vi "传感器测试单片译码器.vi"() -> ()   [LabVIEW 2018]
panel:
  out "缓存":dbl
  out "数值 2":dbl
  out "data 6":bool[](array[boolean]) caption="数据"
  out "初始化的数组 2":dbl[][](array[numeric])
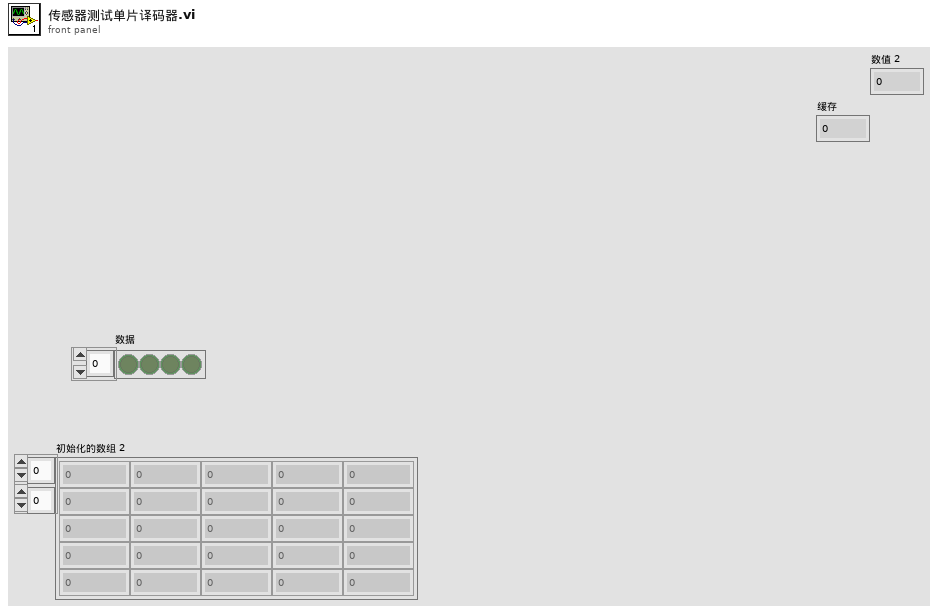
[diagram p1: front panel]
types:
  T1 = enum16{"初始化", "s11", "s12", "s13", "s14", "s15", "s21", "s22", "s23", "s24", "s25", "s31", "s32", "s33", "s34", "s35"}
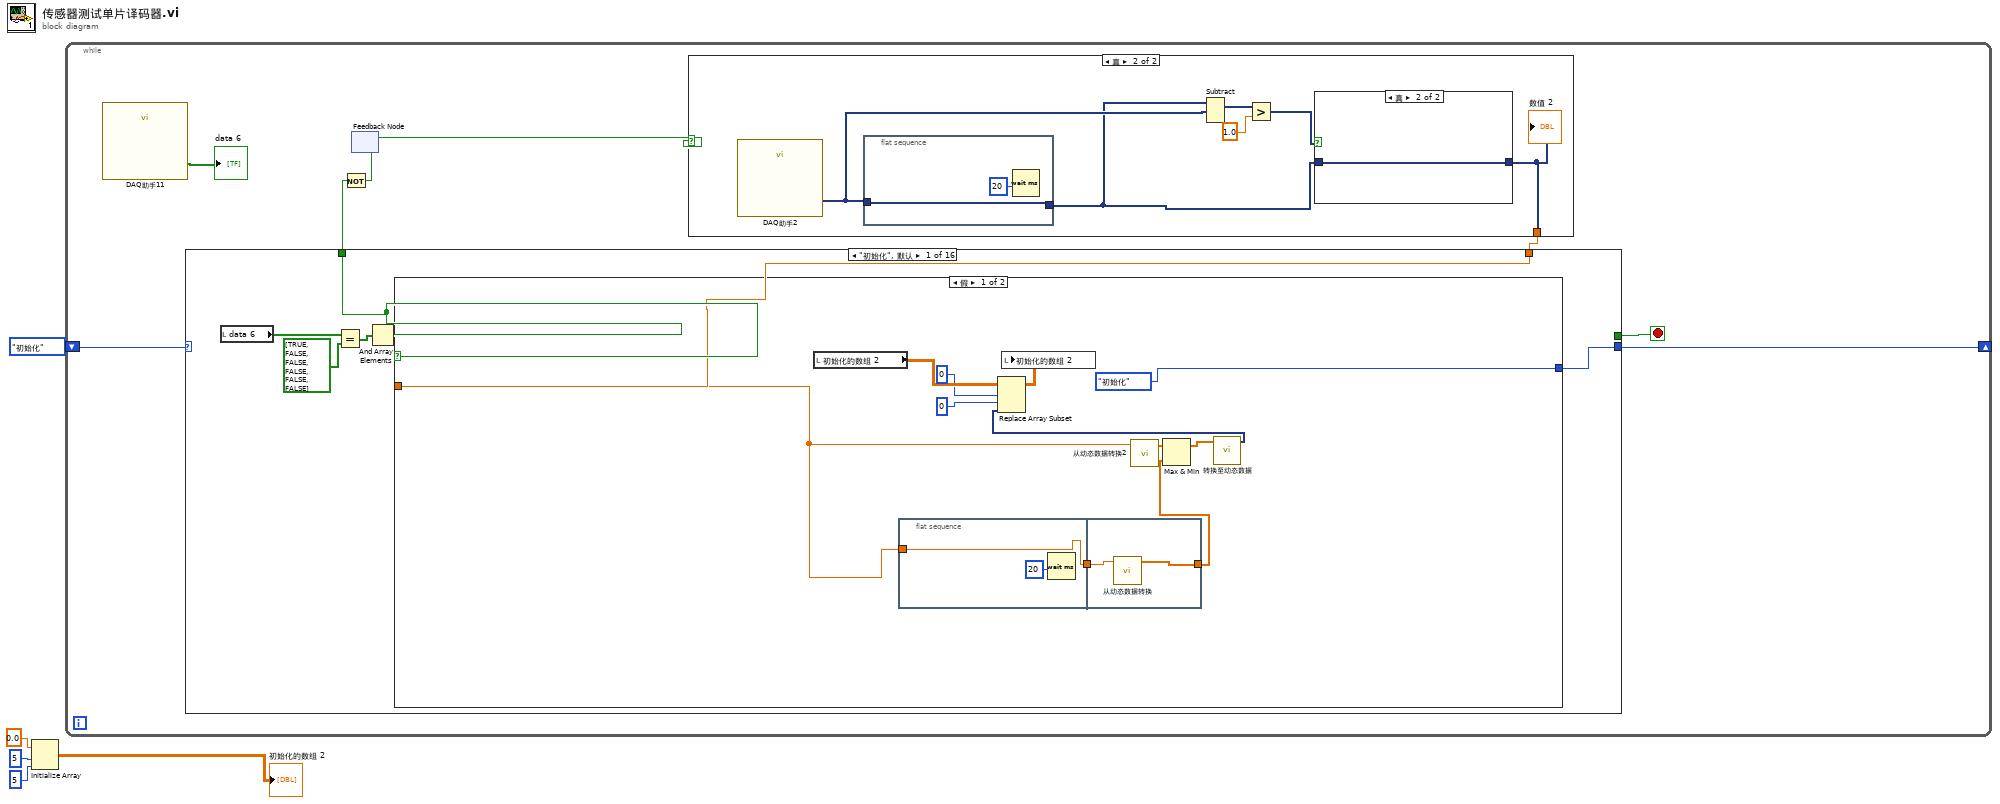
[diagram p0: block diagram]
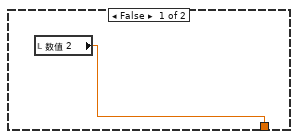
[diagram p2: hidden frame]
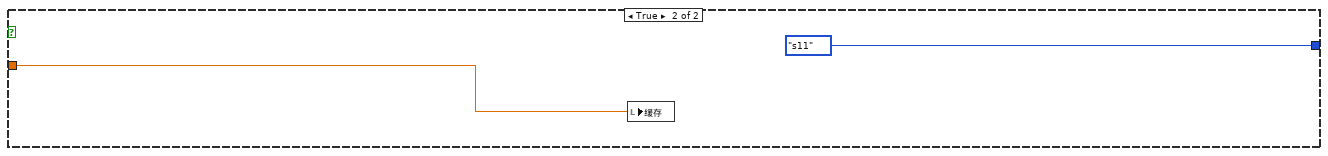
[diagram p4: hidden frame]
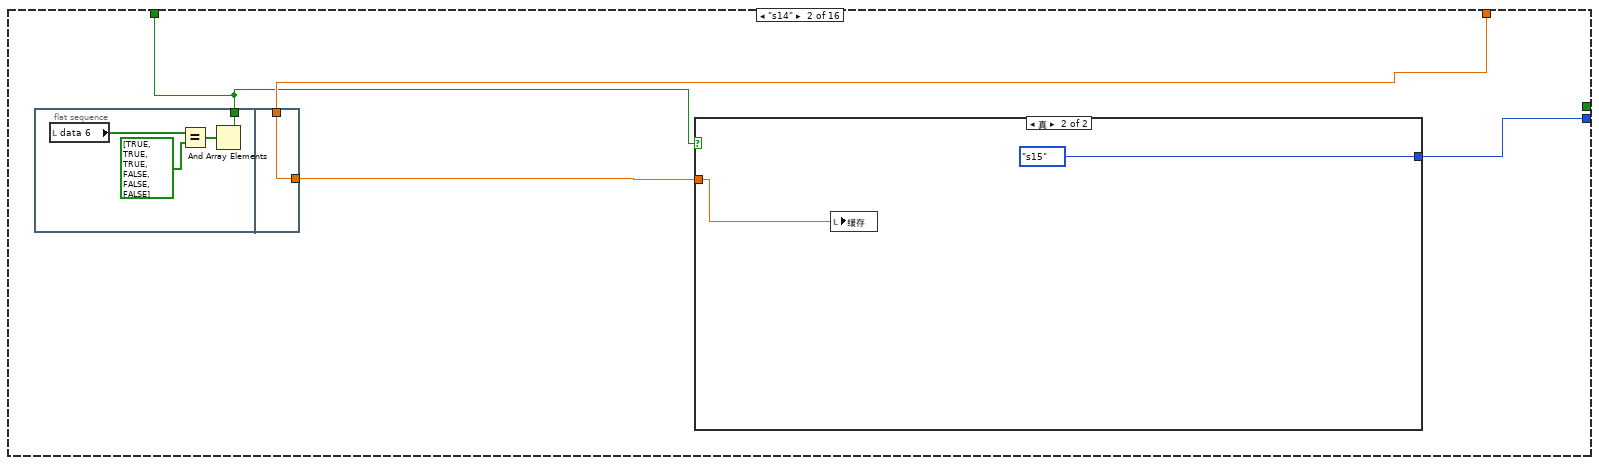
[diagram p5: hidden frame]
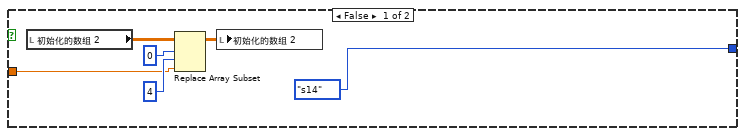
[diagram p6: hidden frame]
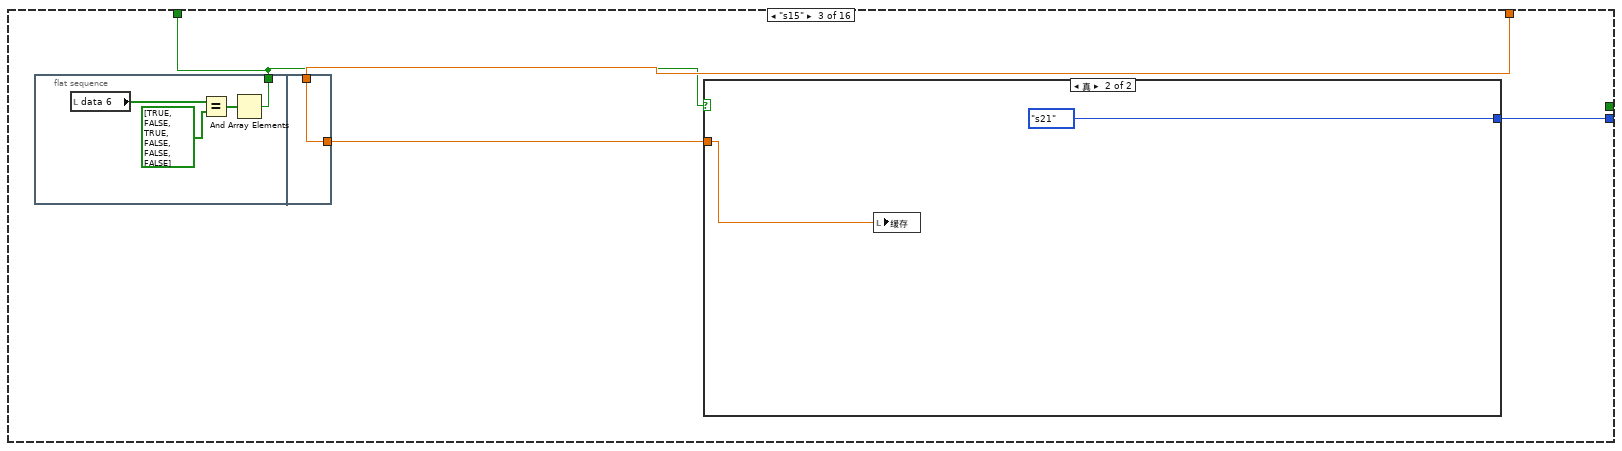
[diagram p7: hidden frame]
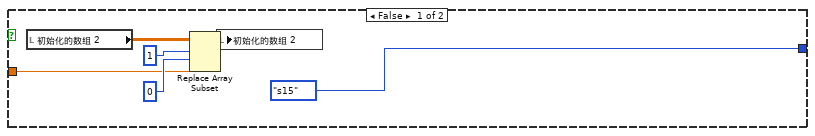
[diagram p8: hidden frame]
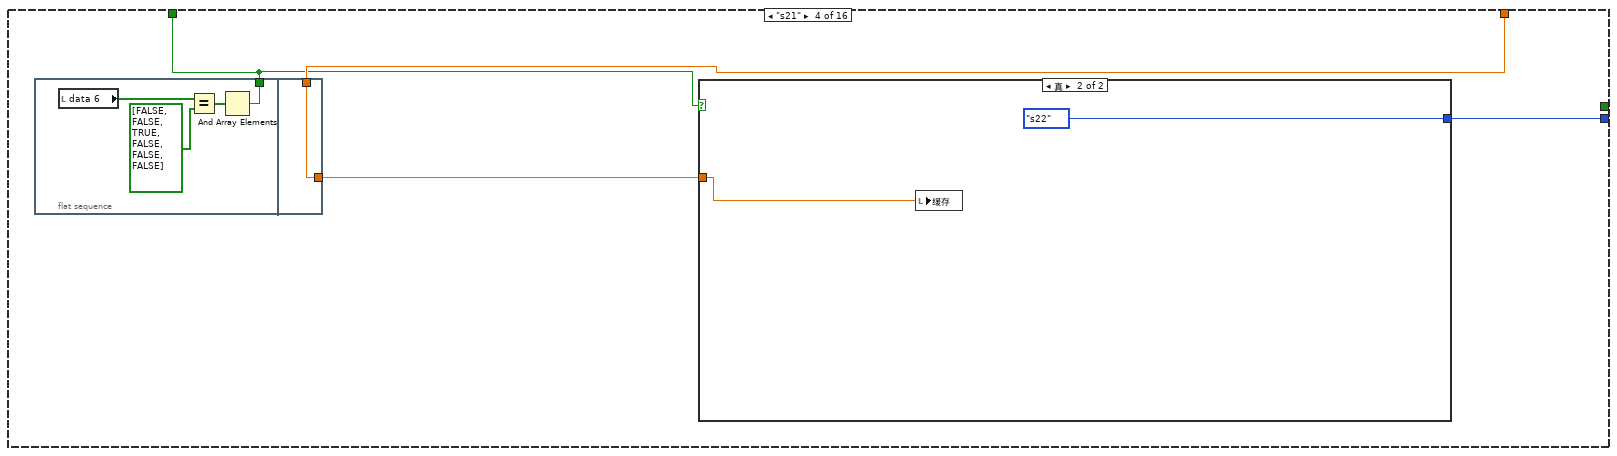
[diagram p9: hidden frame]
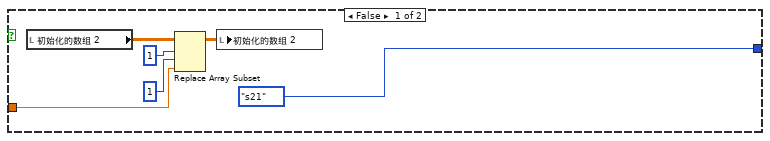
[diagram p10: hidden frame]
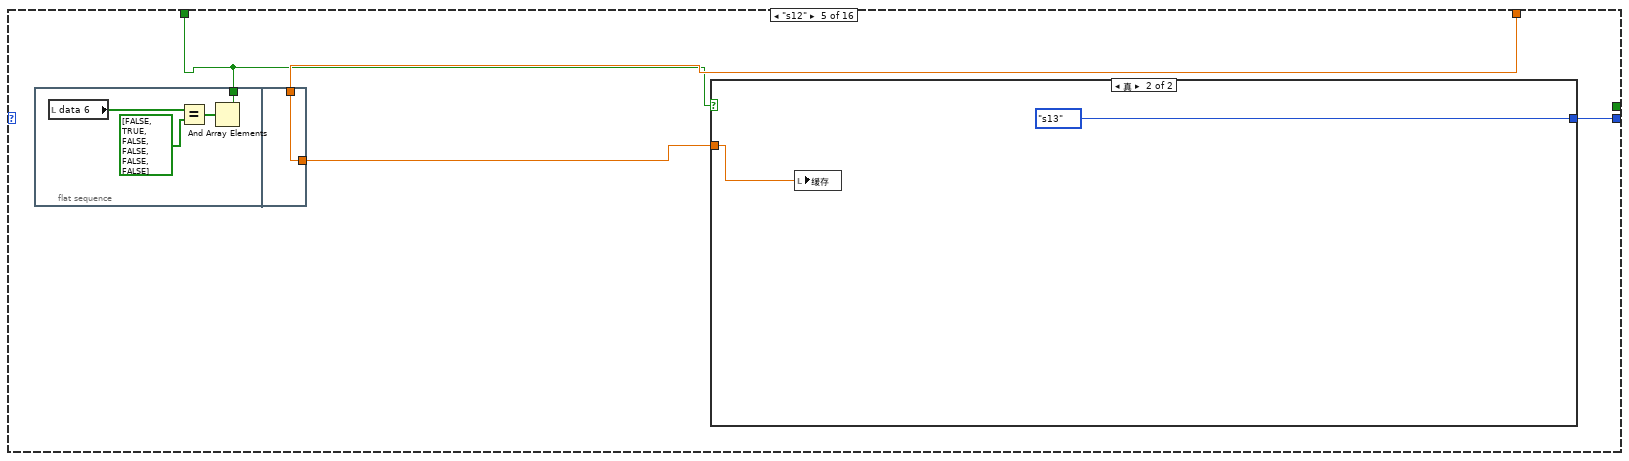
[diagram p11: hidden frame]
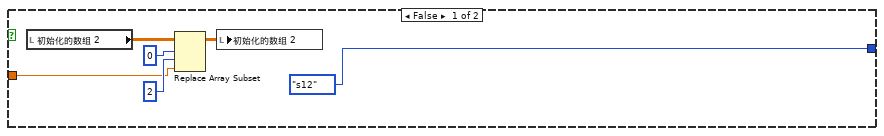
[diagram p12: hidden frame]
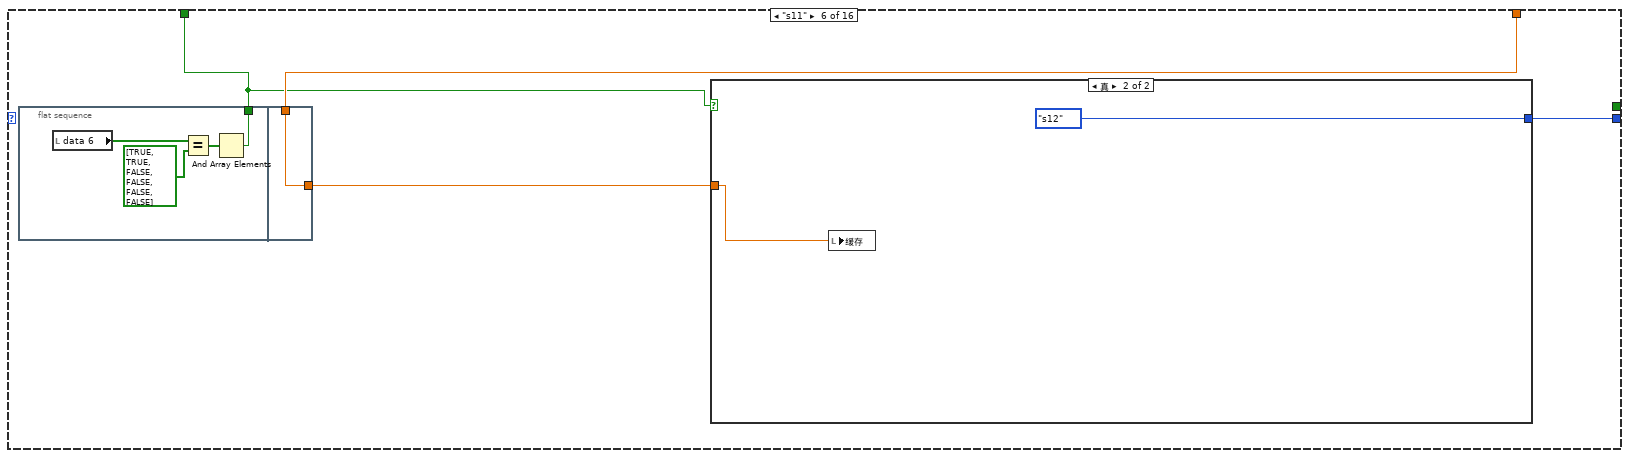
[diagram p13: hidden frame]
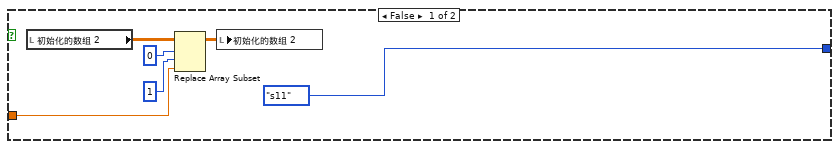
[diagram p14: hidden frame]
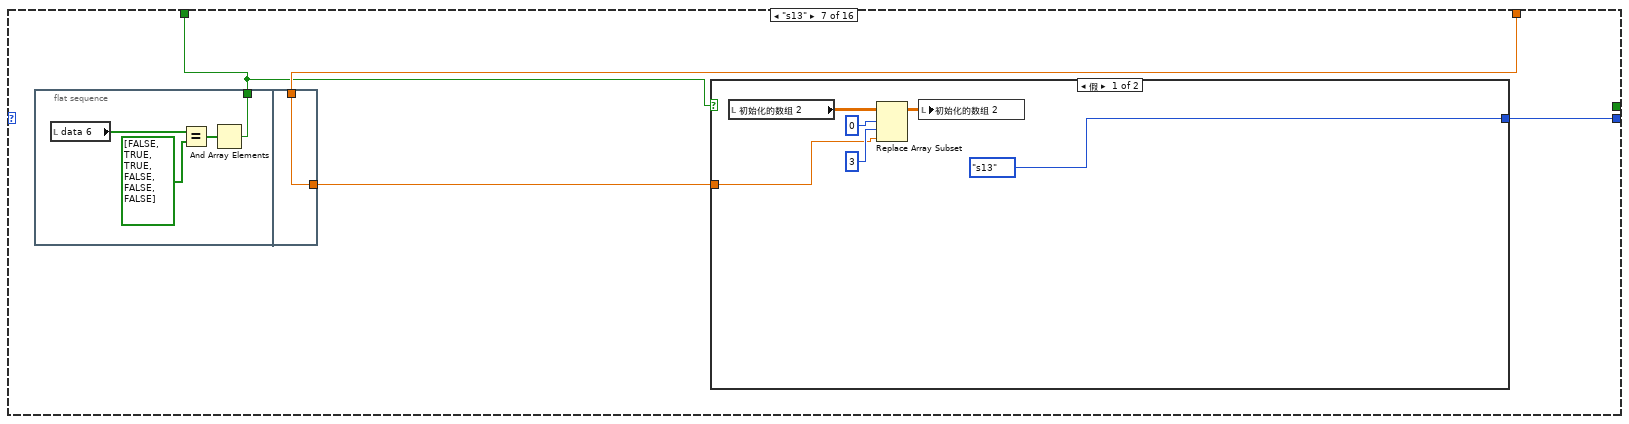
[diagram p15: hidden frame]
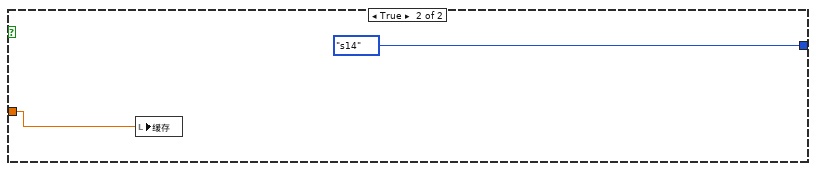
[diagram p16: hidden frame]
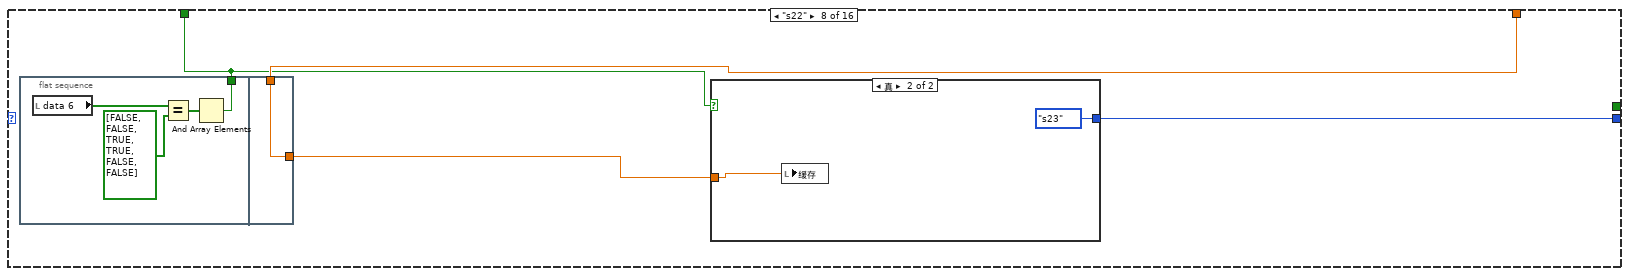
[diagram p17: hidden frame]
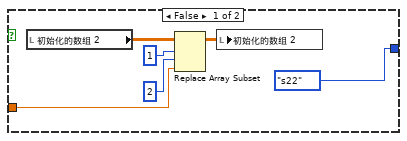
[diagram p18: hidden frame]
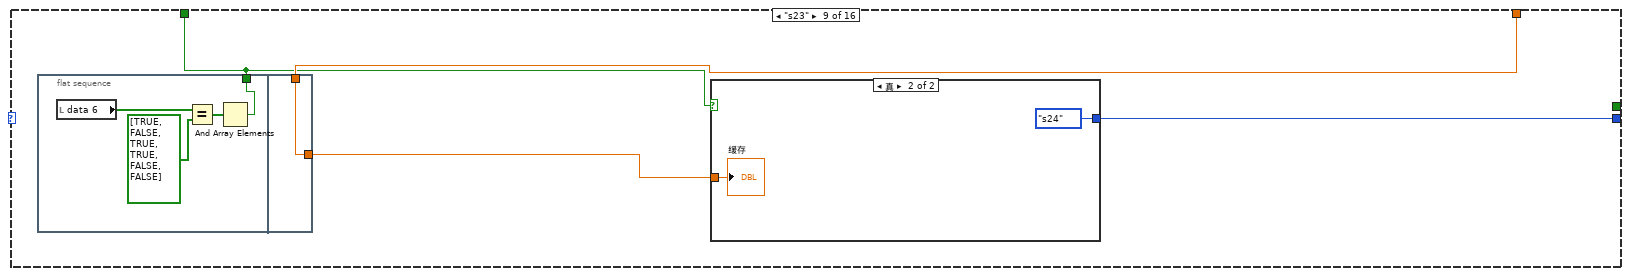
[diagram p19: hidden frame]
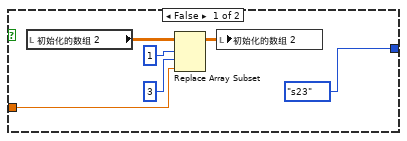
[diagram p20: hidden frame]
diagram:
  n1 = Initialize Array(0.0 ("元素"), 5 ("维数大小"), 5 ("维数大小")) -> (→"初始化的数组 2":dbl[][])
  n2 = while {
    shift-right: [w12] -> _
    shift-left: T1."初始化" ("枚举") -> [w13]
    stop <- w10 stop-if-true
    n3 = call "DAQ助手11"() -> ("data"=→"data 6":bool[])  [unwired: 17 in, 2 out]
    n4 = feedback #1() -> (w6:bool)  [unwired: 1 in]
    n5 = case shown="真" w6 {
      tunnel: [w14 w17] -> w9
      frame False {
        n6 = local read "数值 2"() -> (w14:dbl)
      }
      frame True {
        n7 = call "DAQ助手2"() -> ("data"=w16:dynamicdata)  [unwired: 17 in, 2 out]
        n8 = flat-sequence {
          tunnel: w16 -> [w23]
          tunnel: [w23] -> w15
          frame #0 {
            n9 = Wait (ms)(milliseconds to wait=u32 20 ("毫秒计时值")) -> ()  [unwired: 1 out]
          }
        }
        n10 = Subtract(1:w16, 2:w15) -> (0:w20:dynamicdata)  [unwired: 1 in, 1 out]
        n11 = Greater?(x=w20, y=1.0) -> (0:w18:dynamicdata)
        n12 = case shown="真" w18 {
          tunnel: w15 -> [w21 w22]
          tunnel: [w21 w22] -> w17
          frame False {
          }
          frame True {
          }
        }
        "数值 2" <- w17
      }
    }
    n13 = case shown="\"初始化\", 默认" w13 {
      tunnel: [w30 w51 w68 w85 w102 w119 w136 w153 w170 w187 w204 w221 w238 w255 w272 w291] -> w12
      tunnel: [_ _ _ _ _ _ _ _ _ _ _ _ _ _ _ w292] -> w10
      tunnel: w9 -> [w25 w50 w67 w83 w100 w117 w134 w152 w169 w186 w203 w220 w237 w253 w271 w286]
      tunnel: [w26 w48 w65 w82 w99 w116 w133 w150 w167 w184 w201 w218 w235 w252 w269 w289] -> w8
      frame "初始化", Default {
        n14 = local read "data 6"() -> (w28:bool[])
        n15 = Equal?(x=w28, y=bool[] [TRUE, FALSE, FALSE, FALSE, FALSE, FALSE]) -> (x = y?=w29:bool[])
        n16 = And Array Elements(Boolean array=w29) -> (logical AND=w26:bool)
        n17 = case shown="假" w26 {
          tunnel: [T1."初始化" ("枚举") T1."s11" ("枚举")] -> w30
          tunnel: w25 -> [w31 w46]
          frame False {
            n18 = local read "初始化的数组 2"() -> (w41:dbl[][])
            n19 = flat-sequence {
              tunnel: [w42] -> w32
              tunnel: w31 -> [w42]
              tunnel: [w45] -> w36
              tunnel: w32 -> [w44]
              frame #0 {
                n20 = Wait (ms)(milliseconds to wait=u32 20 ("毫秒计时值")) -> ()  [unwired: 1 out]
              }
              frame #1 {
                n21 = call "从动态数据转换"("Dynamic Data Type"=w44) -> ("Array"=w45:dbl[])  [unwired: 3 in]
              }
            }
            n22 = call "从动态数据转换2"("Dynamic Data Type"=w31) -> ("Array"=w35:dbl[])  [unwired: 3 in]
            n23 = Max & Min(x=w35, y=w36) -> (max(x,y)=w34:dbl[])  [unwired: 1 out]
            n24 = call "转换至动态数据"("Array"=w34) -> ("Dynamic Data Type"=w33:dynamicdata)  [unwired: 3 in]
            n25 = Replace Array Subset(array=w41, new element=w33, index (row)=0 ("禁用的索引 (行)"), index (col)=0 ("禁用的索引 (列)")) -> (w38:dbl[][])
            n26 = local write "初始化的数组 2"(w38) -> ()
          }
          frame True {
            n27 = local write "缓存"(w46) -> ()
          }
        }
      }
      frame "s14" {
        n28 = flat-sequence {
          tunnel: [w52] -> w48
          tunnel: w50 -> [w56]
          tunnel: [w56] -> w49
          frame #0 {
            n29 = local read "data 6"() -> (w55:bool[])
            n30 = Equal?(x=w55, y=bool[] [TRUE, TRUE, TRUE, FALSE, FALSE, FALSE]) -> (x = y?=w54:bool[])
            n31 = And Array Elements(Boolean array=w54) -> (logical AND=w52:bool)
          }
          frame #1 {
          }
        }
        n32 = case shown="真" w48 {
          tunnel: [T1."s14" ("枚举") T1."s15" ("枚举")] -> w51
          tunnel: w49 -> [w57 w63]
          frame False {
            n33 = local read "初始化的数组 2"() -> (w61:dbl[][])
            n34 = Replace Array Subset(array=w61, new element=w57, index (row)=0 ("禁用的索引 (行)"), index (col)=4 ("禁用的索引 (列)")) -> (w62:dbl[][])
            n35 = local write "初始化的数组 2"(w62) -> ()
          }
          frame True {
            n36 = local write "缓存"(w63) -> ()
          }
        }
      }
      frame "s15" {
        n37 = flat-sequence {
          tunnel: [w69] -> w65
          tunnel: w67 -> [w73]
          tunnel: [w73] -> w66
          frame #0 {
            n38 = local read "data 6"() -> (w72:bool[])
            n39 = Equal?(x=w72, y=bool[] [TRUE, FALSE, TRUE, FALSE, FALSE, FALSE]) -> (x = y?=w71:bool[])
            n40 = And Array Elements(Boolean array=w71) -> (logical AND=w69:bool)
          }
          frame #1 {
          }
        }
        n41 = case shown="真" w65 {
          tunnel: [T1."s15" ("枚举") T1."s21" ("枚举")] -> w68
          tunnel: w66 -> [w74 w80]
          frame False {
            n42 = local read "初始化的数组 2"() -> (w78:dbl[][])
            n43 = Replace Array Subset(array=w78, new element=w74, index (row)=1 ("禁用的索引 (行)"), index (col)=0 ("禁用的索引 (列)")) -> (w79:dbl[][])
            n44 = local write "初始化的数组 2"(w79) -> ()
          }
          frame True {
            n45 = local write "缓存"(w80) -> ()
          }
        }
      }
      frame "s21" {
        n46 = flat-sequence {
          tunnel: [w86] -> w82
          tunnel: [w90] -> w84
          tunnel: w83 -> [w90]
          frame #0 {
            n47 = local read "data 6"() -> (w89:bool[])
            n48 = Equal?(x=w89, y=bool[] [FALSE, FALSE, TRUE, FALSE, FALSE, FALSE]) -> (x = y?=w88:bool[])
            n49 = And Array Elements(Boolean array=w88) -> (logical AND=w86:bool)
          }
          frame #1 {
          }
        }
        n50 = case shown="真" w82 {
          tunnel: [T1."s21" ("枚举") T1."s22" ("枚举")] -> w85
          tunnel: w84 -> [w91 w97]
          frame False {
            n51 = local read "初始化的数组 2"() -> (w95:dbl[][])
            n52 = Replace Array Subset(array=w95, new element=w91, index (row)=1 ("禁用的索引 (行)"), index (col)=1 ("禁用的索引 (列)")) -> (w96:dbl[][])
            n53 = local write "初始化的数组 2"(w96) -> ()
          }
          frame True {
            n54 = local write "缓存"(w97) -> ()
          }
        }
      }
      frame "s12" {
        n55 = flat-sequence {
          tunnel: [w103] -> w99
          tunnel: w100 -> [w107]
          tunnel: [w107] -> w101
          frame #0 {
            n56 = local read "data 6"() -> (w106:bool[])
            n57 = Equal?(x=w106, y=bool[] [FALSE, TRUE, FALSE, FALSE, FALSE, FALSE]) -> (x = y?=w105:bool[])
            n58 = And Array Elements(Boolean array=w105) -> (logical AND=w103:bool)
          }
          frame #1 {
          }
        }
        n59 = case shown="真" w99 {
          tunnel: [T1."s12" ("枚举") T1."s13" ("枚举")] -> w102
          tunnel: w101 -> [w108 w114]
          frame False {
            n60 = local read "初始化的数组 2"() -> (w112:dbl[][])
            n61 = Replace Array Subset(array=w112, new element=w108, index (row)=0 ("禁用的索引 (行)"), index (col)=2 ("禁用的索引 (列)")) -> (w113:dbl[][])
            n62 = local write "初始化的数组 2"(w113) -> ()
          }
          frame True {
            n63 = local write "缓存"(w114) -> ()
          }
        }
      }
      frame "s11" {
        n64 = flat-sequence {
          tunnel: [w120] -> w116
          tunnel: [w124] -> w118
          tunnel: w117 -> [w124]
          frame #0 {
            n65 = local read "data 6"() -> (w122:bool[])
            n66 = Equal?(x=w122, y=bool[] [TRUE, TRUE, FALSE, FALSE, FALSE, FALSE]) -> (x = y?=w123:bool[])
            n67 = And Array Elements(Boolean array=w123) -> (logical AND=w120:bool)
          }
          frame #1 {
          }
        }
        n68 = case shown="真" w116 {
          tunnel: [T1."s11" ("枚举") T1."s12" ("枚举")] -> w119
          tunnel: w118 -> [w125 w131]
          frame False {
            n69 = local read "初始化的数组 2"() -> (w130:dbl[][])
            n70 = Replace Array Subset(array=w130, new element=w125, index (row)=0 ("禁用的索引 (行)"), index (col)=1 ("禁用的索引 (列)")) -> (w127:dbl[][])
            n71 = local write "初始化的数组 2"(w127) -> ()
          }
          frame True {
            n72 = local write "缓存"(w131) -> ()
          }
        }
      }
      frame "s13" {
        n73 = flat-sequence {
          tunnel: [w137] -> w133
          tunnel: [w141] -> w135
          tunnel: w134 -> [w141]
          frame #0 {
            n74 = local read "data 6"() -> (w140:bool[])
            n75 = Equal?(x=w140, y=bool[] [FALSE, TRUE, TRUE, FALSE, FALSE, FALSE]) -> (x = y?=w139:bool[])
            n76 = And Array Elements(Boolean array=w139) -> (logical AND=w137:bool)
          }
          frame #1 {
          }
        }
        n77 = case shown="假" w133 {
          tunnel: [T1."s13" ("枚举") T1."s14" ("枚举")] -> w136
          tunnel: w135 -> [w142 w148]
          frame False {
            n78 = local read "初始化的数组 2"() -> (w146:dbl[][])
            n79 = Replace Array Subset(array=w146, new element=w142, index (row)=0 ("禁用的索引 (行)"), index (col)=3 ("禁用的索引 (列)")) -> (w147:dbl[][])
            n80 = local write "初始化的数组 2"(w147) -> ()
          }
          frame True {
            n81 = local write "缓存"(w148) -> ()
          }
        }
      }
      frame "s22" {
        n82 = flat-sequence {
          tunnel: [w154] -> w150
          tunnel: w152 -> [w158]
          tunnel: [w158] -> w151
          frame #0 {
            n83 = local read "data 6"() -> (w156:bool[])
            n84 = Equal?(x=w156, y=bool[] [FALSE, FALSE, TRUE, TRUE, FALSE, FALSE]) -> (x = y?=w157:bool[])
            n85 = And Array Elements(Boolean array=w157) -> (logical AND=w154:bool)
          }
          frame #1 {
          }
        }
        n86 = case shown="真" w150 {
          tunnel: [T1."s22" ("枚举") T1."s23" ("枚举")] -> w153
          tunnel: w151 -> [w159 w165]
          frame False {
            n87 = local read "初始化的数组 2"() -> (w163:dbl[][])
            n88 = Replace Array Subset(array=w163, new element=w159, index (row)=1 ("禁用的索引 (行)"), index (col)=2 ("禁用的索引 (列)")) -> (w164:dbl[][])
            n89 = local write "初始化的数组 2"(w164) -> ()
          }
          frame True {
            n90 = local write "缓存"(w165) -> ()
          }
        }
      }
      frame "s23" {
        n91 = flat-sequence {
          tunnel: [w171] -> w167
          tunnel: w169 -> [w175]
          tunnel: [w175] -> w168
          frame #0 {
            n92 = local read "data 6"() -> (w173:bool[])
            n93 = Equal?(x=w173, y=bool[] [TRUE, FALSE, TRUE, TRUE, FALSE, FALSE]) -> (x = y?=w174:bool[])
            n94 = And Array Elements(Boolean array=w174) -> (logical AND=w171:bool)
          }
          frame #1 {
          }
        }
        n95 = case shown="真" w167 {
          tunnel: [T1."s23" ("枚举") T1."s24" ("枚举")] -> w170
          tunnel: w168 -> [w176 w182]
          frame False {
            n96 = local read "初始化的数组 2"() -> (w180:dbl[][])
            n97 = Replace Array Subset(array=w180, new element=w176, index (row)=1 ("禁用的索引 (行)"), index (col)=3 ("禁用的索引 (列)")) -> (w181:dbl[][])
            n98 = local write "初始化的数组 2"(w181) -> ()
          }
          frame True {
            "缓存" <- w182
          }
        }
      }
      frame "s24" {
        n99 = flat-sequence {
          tunnel: [w188] -> w184
          tunnel: w186 -> [w192]
          tunnel: [w192] -> w185
          frame #0 {
            n100 = local read "data 6"() -> (w190:bool[])
            n101 = Equal?(x=w190, y=bool[] [TRUE, TRUE, TRUE, TRUE, FALSE, FALSE]) -> (x = y?=w191:bool[])
            n102 = And Array Elements(Boolean array=w191) -> (logical AND=w188:bool)
          }
          frame #1 {
          }
        }
        n103 = case shown="真" w184 {
          tunnel: [T1."s24" ("枚举") T1."s25" ("枚举")] -> w187
          tunnel: w185 -> [w193 w199]
          frame False {
            n104 = local read "初始化的数组 2"() -> (w196:dbl[][])
            n105 = Replace Array Subset(array=w196, new element=w193, index (row)=1 ("禁用的索引 (行)"), index (col)=4 ("禁用的索引 (列)")) -> (w195:dbl[][])
            n106 = local write "初始化的数组 2"(w195) -> ()
          }
          frame True {
            n107 = local write "缓存"(w199) -> ()
          }
        }
      }
      frame "s25" {
        n108 = flat-sequence {
          tunnel: [w205] -> w201
          tunnel: w203 -> [w209]
          tunnel: [w209] -> w202
          frame #0 {
            n109 = local read "data 6"() -> (w207:bool[])
            n110 = Equal?(x=w207, y=bool[] [FALSE, TRUE, TRUE, TRUE, FALSE, FALSE]) -> (x = y?=w208:bool[])
            n111 = And Array Elements(Boolean array=w208) -> (logical AND=w205:bool)
          }
          frame #1 {
          }
        }
        n112 = case shown="真" w201 {
          tunnel: [T1."s25" ("枚举") T1."s31" ("枚举")] -> w204
          tunnel: w202 -> [w210 w216]
          frame False {
            n113 = local read "初始化的数组 2"() -> (w213:dbl[][])
            n114 = Replace Array Subset(array=w213, new element=w210, index (row)=2 ("禁用的索引 (行)"), index (col)=0 ("禁用的索引 (列)")) -> (w212:dbl[][])
            n115 = local write "初始化的数组 2"(w212) -> ()
          }
          frame True {
            n116 = local write "缓存"(w216) -> ()
          }
        }
      }
      frame "s31" {
        n117 = flat-sequence {
          tunnel: [w222] -> w218
          tunnel: w220 -> [w226]
          tunnel: [w226] -> _
          tunnel: [w226] -> w219
          frame #0 {
            n118 = local read "data 6"() -> (w224:bool[])
            n119 = Equal?(x=w224, y=bool[] [FALSE, TRUE, FALSE, TRUE, FALSE, FALSE]) -> (x = y?=w225:bool[])
            n120 = And Array Elements(Boolean array=w225) -> (logical AND=w222:bool)
          }
          frame #1 {
          }
        }
        n121 = case shown="真" w218 {
          tunnel: [T1."s31" ("枚举") T1."s32" ("枚举")] -> w221
          tunnel: w219 -> [w227 w233]
          frame False {
            n122 = local read "初始化的数组 2"() -> (w230:dbl[][])
            n123 = Replace Array Subset(array=w230, new element=w227, index (row)=2 ("禁用的索引 (行)"), index (col)=1 ("禁用的索引 (列)")) -> (w229:dbl[][])
            n124 = local write "初始化的数组 2"(w229) -> ()
          }
          frame True {
            n125 = local write "缓存"(w233) -> ()
          }
        }
      }
      frame "s32" {
        n126 = flat-sequence {
          tunnel: [w239] -> w235
          tunnel: [w243] -> w236
          tunnel: w237 -> [w243]
          frame #0 {
            n127 = local read "data 6"() -> (w241:bool[])
            n128 = Equal?(x=w241, y=bool[] [TRUE, TRUE, FALSE, TRUE, FALSE, FALSE]) -> (x = y?=w242:bool[])
            n129 = And Array Elements(Boolean array=w242) -> (logical AND=w239:bool)
          }
          frame #1 {
          }
        }
        n130 = case shown="真" w235 {
          tunnel: [T1."s32" ("枚举") T1."s33" ("枚举")] -> w238
          tunnel: w236 -> [w244 w250]
          frame False {
            n131 = local read "初始化的数组 2"() -> (w247:dbl[][])
            n132 = Replace Array Subset(array=w247, new element=w244, index (row)=2 ("禁用的索引 (行)"), index (col)=2 ("禁用的索引 (列)")) -> (w246:dbl[][])
            n133 = local write "初始化的数组 2"(w246) -> ()
          }
          frame True {
            n134 = local write "缓存"(w250) -> ()
          }
        }
      }
      frame "s33" {
        n135 = flat-sequence {
          tunnel: [w256] -> w252
          tunnel: [w260] -> w254
          tunnel: w253 -> [w260]
          frame #0 {
            n136 = local read "data 6"() -> (w258:bool[])
            n137 = Equal?(x=w258, y=bool[] [TRUE, FALSE, FALSE, TRUE, FALSE, FALSE]) -> (x = y?=w259:bool[])
            n138 = And Array Elements(Boolean array=w259) -> (logical AND=w256:bool)
          }
          frame #1 {
          }
        }
        n139 = case shown="真" w252 {
          tunnel: [T1."s33" ("枚举") T1."s34" ("枚举")] -> w255
          tunnel: w254 -> [w261 w267]
          frame False {
            n140 = local read "初始化的数组 2"() -> (w264:dbl[][])
            n141 = Replace Array Subset(array=w264, new element=w261, index (row)=2 ("禁用的索引 (行)"), index (col)=3 ("禁用的索引 (列)")) -> (w263:dbl[][])
            n142 = local write "初始化的数组 2"(w263) -> ()
          }
          frame True {
            n143 = local write "缓存"(w267) -> ()
          }
        }
      }
      frame "s34" {
        n144 = flat-sequence {
          tunnel: [w273] -> w269
          tunnel: w271 -> [w277]
          tunnel: [w277] -> w270
          frame #0 {
            n145 = local read "data 6"() -> (w275:bool[])
            n146 = Equal?(x=w275, y=bool[] [FALSE, FALSE, FALSE, TRUE, FALSE, FALSE]) -> (x = y?=w276:bool[])
            n147 = And Array Elements(Boolean array=w276) -> (logical AND=w273:bool)
          }
          frame #1 {
          }
        }
        n148 = case shown="真" w269 {
          tunnel: [T1."s34" ("枚举") T1."s35" ("枚举")] -> w272
          tunnel: w270 -> [w278 w284]
          frame False {
            n149 = local read "初始化的数组 2"() -> (w281:dbl[][])
            n150 = Replace Array Subset(array=w281, new element=w278, index (row)=2 ("禁用的索引 (行)"), index (col)=4 ("禁用的索引 (列)")) -> (w280:dbl[][])
            n151 = local write "初始化的数组 2"(w280) -> ()
          }
          frame True {
            n152 = local write "缓存"(w284) -> ()
          }
        }
      }
      frame "s35" {
        n153 = flat-sequence {
          tunnel: [w294] -> w288
          tunnel: [w293] -> w287
          tunnel: [w298] -> w289
          tunnel: w288 -> [w298]
          tunnel: [w297] -> w290
          tunnel: w287 -> [_]
          tunnel: w286 -> [w297]
          frame #0 {
            n154 = local read "data 6"() -> (w296:bool[])
            n155 = Equal?(x=w296, y=bool[] [FALSE, FALSE, FALSE, FALSE, FALSE, FALSE]) -> (x = y?=w293:bool[])
            n156 = And Array Elements(Boolean array=w293) -> (logical AND=w294:bool)
          }
          frame #1 {
          }
        }
        n157 = case shown="真" w289 {
          tunnel: [_ TRUE] -> w292
          tunnel: [T1."s35" ("枚举") T1."s35" ("枚举")] -> w291
          tunnel: w290 -> [w299 w305]
          frame False {
            n158 = local read "初始化的数组 2"() -> (w302:dbl[][])
            n159 = Replace Array Subset(array=w302, new element=w299, index (row)=3 ("禁用的索引 (行)"), index (col)=0 ("禁用的索引 (列)")) -> (w301:dbl[][])
            n160 = local write "初始化的数组 2"(w301) -> ()
          }
          frame True {
            n161 = local write "缓存"(w305) -> ()
          }
        }
      }
    }
    n162 = Not(x=w8) -> (.not. x?=w7:bool)
    n163 = feedback-in #1(w7) -> ()
  }
